vi "Trial v6.vi"(2 "error in (no error)":errorcluster, 3 "queue in":refnum<queue>, 4 "DDA":bool=TRUE) -> (0 "error out":errorcluster, 1 "queue out":refnum<queue>)   [LabVIEW 2017]
uses:
  <vilib>/Analysis/_algsub.llb/Real Vector Norm.vi
  <vilib>/Analysis/baseanly.llb/Real A x B.vi
  <vilib>/Analysis/baseanly.llb/Real Dot Product.vi
  <vilib>/Analysis/baseanly.llb/Outer Product.vi
  <vilib>/Analysis/baseanly.llb/Real Outer Product.vi
  <vilib>/robotics/Kinematics/Create Lie Group Matrix.vi
  SubVI/Global.vi
  <vilib>/Analysis/7linalg.llb/Create Special Matrix.vi
  <vilib>/Analysis/7linalg.llb/Create Special Real Matrix.vi
  <vilib>/Analysis/Matrix/Numeric/Multiply/Multiply.vi
  <vilib>/Analysis/Matrix/Numeric/Multiply/Multiply - RM,R.vi
  <vilib>/Analysis/Matrix/Numeric/Multiply/Multiply - R,RM.vi
  <vilib>/Analysis/Matrix/Numeric/Add/Add.vi
  <vilib>/Analysis/Matrix/Numeric/Add/Add - RM,RM.vi
  Control/Damping.ctl
  <vilib>/robotics/Kinematics/NI_Kinematics.lvlib
  <vilib>/Analysis/NI_AALBase.lvlib
  <vilib>/Analysis/NI_AALPro.lvlib
panel:
  in  "ACTION":dbl[](array[numeric])=[1.0, 0.5, -0.5, -1.0]
  in  "DELTAx":dbl=0.01
  in  "Algorithm Parameter":T1={"alpha Rbar"=0.1, "lambda w"=0.99, "lambda theta"=0.99, "alpha w"=0.1, "alpha theta"=0.1} {"alpha theta" scale=0.0..1.0; "alpha w" scale=0.0..1.0; "lambda theta" scale=0.0..1.0; "lambda w" scale=0.0..1.0; "alpha Rbar" scale=0.0..1.0}
  in  "Basis":enum16{"Polynomial", "Fourier"}(ring)
  in  "n":i32=2
  out "Guide":bool
  in  "DDA Wait (ms)":u32=1000
  in  "epsilon (deg)":dbl=5.0
  in  "Omega (deg/s)":dbl=10.0
  in  "Trial Wait (ms)":u32=10
  in  "RoM (deg)":dbl=75.0 format="%#_13g"
  out "Variable":T2={"state"=[1.0, 0.029510106398225495, 0.7899999999999947], "state'"=[1.0, 0.029510106398225495, 0.7899999999999947], "w"=[-0.776760178088027, 0.02290847510201797, -0.776760178088027, 0.0039017617832994905, -0.032305900148233264, 0.0039017617832994905, -0.008811939810442246, 0.006128296774504617, -0.008811939810442246, 0.08141039795404857, 0.024694708282895942, 0.08141039795404857, 0.000818616387278701, 0.013811079508305709, 0.000818616387278701, 0.007297971648903151, 0.00012749513787888267, 0.007297971648903151, 0.04749276911722675, 0.0020428849734649714, 0.04749276911722675, -0.0005749430419034135, 0.009106369563891898, -0.0005749430419034135, 0.004440396759161163, -0.00026837014810894707, 0.004440396759161163], "zw"=[46.90944570448865, 0.19066468600195396, 46.90944570448865, -0.7931005098682211, 5.860142075356345, -0.7931005098682211, 2.7017068020466164, -0.27486059004893465, 2.7017068020466164, 16.93934246409302, -0.551912667218565, 16.93934246409302, -0.5655566099588606, 2.5899820994142524, -0.5655566099588606, 1.2460084406100564, -0.1713251360039408, 1.2460084406100564, 9.289011953386677, -0.47204075792696587, 9.289011953386677, -0.4122416203188374, 1.437667453855831, -0.4122416203188374, 0.7051975708183595, -0.13015957998160824, 0.7051975708183595], "theta"=[1.4914571304587486e-15, 7.444904250698107e-17, 1.4914571304587486e-15, -4.739219774861162e-16, 6.634247906152909e-16, -4.739219774861162e-16, 7.576246728345865e-17, -1.7431691862520748e-17, 7.576246728345865e-17, 6.558028522386373e-17, 5.693079546893576e-16, 6.558028522386373e-17, 3.990875526750827e-17, -3.9273504773765236e-17, 3.990875526750827e-17, 2.459332078486038e-18, 1.1844914586165022e-17, 2.459332078486038e-18, 1.6785560810690787e-17, 4.0992884372049907e-17, 1.6785560810690787e-17, 1.547195777204608e-17, -1.8245201415855317e-17, 1.547195777204608e-17, 2.728657325438036e-18, -1.5522560327373708e-18, 2.728657325438036e-18, 25.646102280776066, 16.99493096232432, 25.646102280776066, 3.4822002128803744, 1.8527275230967626, 3.4822002128803744, 0.47573357341205397, 0.21371320352095907, 0.47573357341205397, -0.5264282474235465, -0.5422694989375832, -0.5264282474235465, -0.06394125843286388, -0.06344726999994278, -0.06394125843286388, -0.007905815409065703, -0.008246766308638343, -0.007905815409065703, 0.016635359284166797, 0.01856234594691108, 0.016635359284166797, 0.0019481630383850373, 0.0019346346383257145, 0.0019481630383850373, 0.00022262613770425934, 0.0002462738805832368, 0.00022262613770425934, -15.883327960756356, -27.94126620796533, -15.883327960756356, -1.4668314615111306, -3.9624707541982542, -1.4668314615111306, -0.1616174346023939, -0.5356497273885115, -0.1616174346023939, 0.5812202773533058, 0.5336991802087973, 0.5812202773533058, 0.06450129455154789, 0.06598340428988386, 0.06450129455154789, 0.008688278747498104, 0.007665438304981554, 0.008688278747498104, -0.021645624159105748, -0.015864851158712733, -0.021645624159105748, -0.0019966454372759715, -0.002037241101393498, -0.0019966454372759715, -0.0002749105366125961, -0.00020396807290514954, -0.0002749105366125961], "ztheta"=[7.054061451920969e-17, -3.9587003301846824e-16, 7.054061451920969e-17, 6.735802826201208e-18, -4.6286977384745565e-17, 6.735802826201208e-18, 1.393348122000214e-17, -2.2778836767459474e-17, 1.393348122000214e-17, -1.320687697955934e-16, 4.010916693070787e-17, -1.320687697955934e-16, -3.0638380335155074e-17, 3.0483525341288226e-17, -3.0638380335155074e-17, 1.0341705245027453e-17, -1.2480413093924516e-17, 1.0341705245027453e-17, 2.89630956686208e-17, -3.801392344852731e-17, 2.89630956686208e-17, 2.423591043688077e-17, -2.3809460948435052e-17, 2.423591043688077e-17, 4.616160753220477e-18, -4.795459759566049e-18, 4.616160753220477e-18, -2.910976576435246, -1.923969710656085, -2.910976576435246, -0.3974772560222368, -0.2077962325162933, -0.3974772560222368, -0.054121648119702236, -0.024130482735325663, -0.054121648119702236, 0.059512355276425906, 0.06158016230321163, 0.059512355276425906, 0.007261479780099875, 0.007188638739252933, 0.007261479780099875, 0.0008936446993227526, 0.0009399166521141767, 0.0008936446993227526, -0.0018547408233615288, -0.0021286028828297597, -0.0018547408233615288, -0.00022180803768472273, -0.0002182870264243828, -0.00022180803768472273, -2.4785505426840216e-05, -2.841860420413458e-05, -2.4785505426840216e-05, 1.8080184700730275, 3.160240158328639, 1.8080184700730275, 0.16194822643111972, 0.45396056921070077, 0.16194822643111972, 0.01843165528111534, 0.06070135065256019, 0.01843165528111534, -0.0662462980572756, -0.06004323366484613, -0.0662462980572756, -0.007289851049687639, -0.007508393437731105, -0.007289851049687639, -0.000997466379730686, -0.0008586521896839331, -0.000997466379730686, 0.0025324316646370623, 0.0017108705851870154, 0.0025324316646370623, 0.0002232616330359063, 0.00023382606595410158, 0.0002232616330359063, 3.261164823906294e-05, 2.1712455435348493e-05, 3.261164823906294e-05], "R"=0.34176612385999994, "Rbar"=-0.5362314277071021, "eligibility vector"=[0.0, 0.0, 0.0, 0.0, 0.0, 0.0, 0.0, 0.0, 0.0, 0.0, 0.0, 0.0, 0.0, 0.0, 0.0, 0.0, 0.0, 0.0, 0.0, 0.0, 0.0, 0.0, 0.0, 0.0, 0.0, 0.0, 0.0, 0.0, 0.0, 0.0, 0.0, 0.0, 0.0, 0.0, 0.0, 0.0, 0.0, 0.0, 0.0, 0.0, 0.0, 0.0, 0.0, 0.0, 0.0, 0.0, 0.0, 0.0, 0.0, 0.0, 0.0, 0.0, 0.0, 0.0, 0.0, 0.0, 0.0, 0.0, 0.0, 0.0, 0.0, 0.0, 0.0, 0.0, 0.0, 0.0, 0.0, 0.0, 0.0, 0.0, 0.0, 0.0, 0.0, 0.0, 0.0, 0.0, 0.0, 0.0, 0.0, 0.0, 0.0]} {"eligibility vector" format="%#_6f"; "ztheta" format="%#_6f"; "zw" format="%#_6f"; "Rbar" format="%#_6f"; "R" format="%#_6f"; "theta" format="%#_6f"; "w" format="%#_6f"}
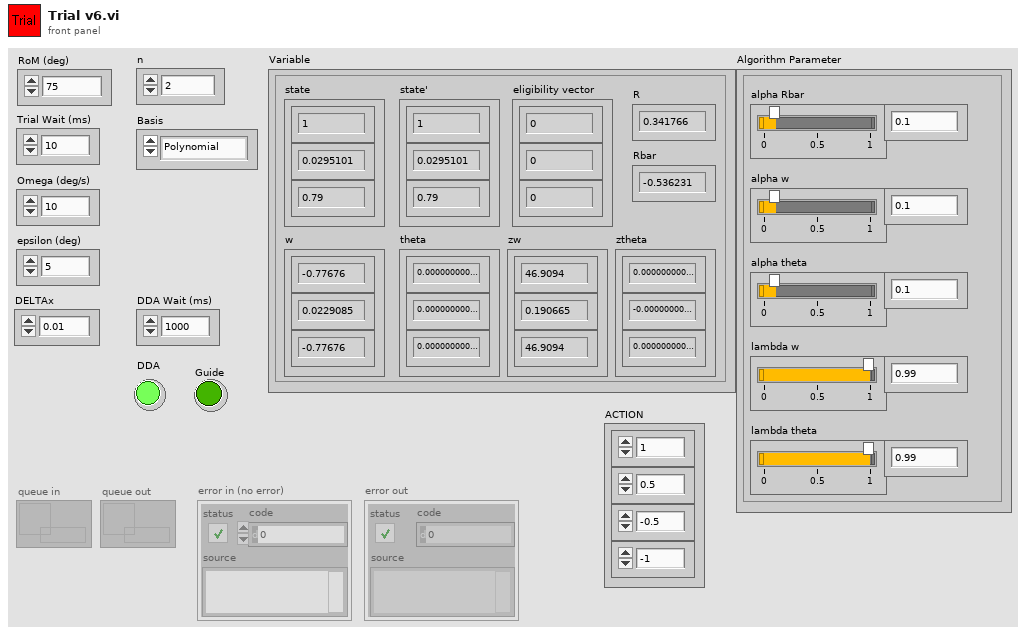
[diagram p1: front panel]
types:
  T1 = cluster{"alpha Rbar":dbl, "lambda w":dbl, "lambda theta":dbl, "alpha w":dbl, "alpha theta":dbl}
  T2 = cluster{"state":dbl[], "state'":dbl[], "w":dbl[], "zw":dbl[], "theta":dbl[], "ztheta":dbl[], "R":dbl, "Rbar":dbl, "eligibility vector":dbl[]}
  T3 = typedef "NI_Matrix.lvlib/RealMatrix.ctl" = dbl[][]
  T4 = typedef "Damping.ctl" = cluster{"Cx":dbl, "Cy":dbl, "Cz":dbl}
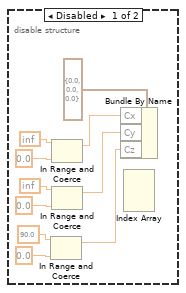
[diagram p2: hidden frame]
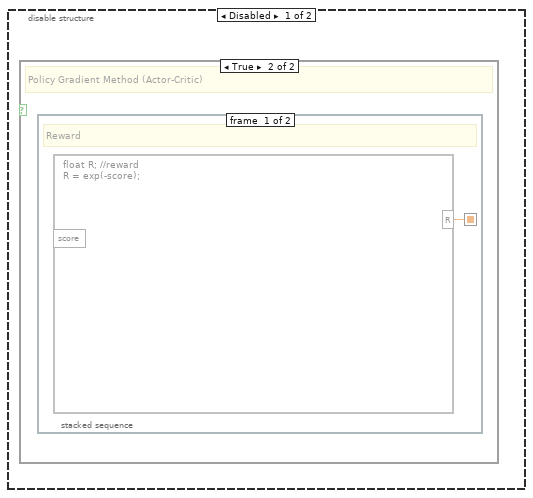
[diagram p3: hidden frame]
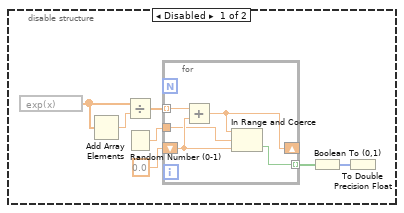
[diagram p6: hidden frame]
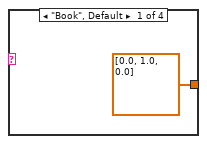
[diagram p9: hidden frame]
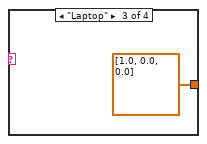
[diagram p10: hidden frame]
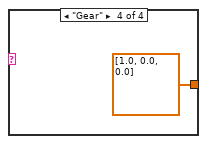
[diagram p11: hidden frame]
diagram:
  n1 = flat-sequence {
    tunnel: "DDA" -> [w11]
    tunnel: "queue in" -> [w10]
    tunnel: "error in (no error)" -> [w9]
    tunnel: [w8] -> w2
    tunnel: [w7] -> w1
    frame #0 {
      n2 = global read "Global.vi" "ADL"() -> (w14:string)
      n3 = case shown="True" w11 {
        tunnel: w10 -> [w16 w32]
        tunnel: w9 -> [w15 w31]
        tunnel: [w15 w29] -> w8
        tunnel: [w16 w30] -> w7
        frame False {
        }
        frame True {
          n4 = call "State.vi"() -> ("state"=w18:dbl[])  [unwired: 11 in]
          n5 = Build Array (concatenate)(w18, 0.0 ("element")) -> (w27:dbl[])
          n6 = call "Feature Vector.vi"("Basis"="Basis", "n"="n", "input"=w18) -> ("feature vector"=w36:dbl[])  [unwired: 8 in]
          n7 = call "Feature Vector.vi"("Basis"="Basis", "n"="n", "input"=w27) -> ("feature vector"=w24:dbl[])  [unwired: 8 in]
          n8 = Array Size(array=w36) -> (size(s)=w35:i32)
          n9 = Array Size(array=w24) -> (size(s)=w23:i32)
          n10 = Initialize Array(0.0 ("element"), w35) -> (w26:dbl[])
          n11 = Initialize Array(0.0 ("element"), w23) -> (w22:dbl[])
          n12 = Bundle By Name(cluster=T2 {"state"=[0.0, 0.0, 0.0], "state'"=[0.0, 0.0, 0.0], "w"=[0.0], "zw"=[0.0], "theta"=[0.0], "ztheta"=[0.0], "R"=0.0, "Rbar"=0.0, "eligibility vector"=[0.0]} ("Variable"), "state"=w18, "w"=w26, "zw"=w26, "theta"=w22, "ztheta"=w22, "Rbar"=0.0) -> (w19:T2)
          n13 = while {
            shift-right: [w38] -> _
            shift-left: w19 -> [w37]
            shift-right: [w42] -> w30
            shift-left: w32 -> [w44]
            shift-right: [w41] -> w29
            shift-left: w31 -> [w43]
            tunnel: "n" -> [w40]
            tunnel: "Basis" -> [w39]
            stop <- w46 stop-if-true
            n14 = local read "Guide"() -> (w45:bool)
            n15 = case shown="True" w45 {
              tunnel: w37 -> [w47 w60]
              tunnel: w44 -> [w49 w67]
              tunnel: w43 -> [w48 w66]
              tunnel: [w49 w65] -> w42
              tunnel: [w48 w64] -> w41
              tunnel: w40 -> [_ w62]
              tunnel: w39 -> [_ w61]
              tunnel: [w47 w56] -> w38
              frame False {
              }
              frame True {
                n16 = flat-sequence {
                  tunnel: w62 -> [w69]
                  tunnel: w61 -> [w68]
                  tunnel: w60 -> [w83]
                  tunnel: [w71] -> w59
                  tunnel: [w69] -> w53
                  tunnel: [w68] -> w50
                  tunnel: w59 -> [w113]
                  tunnel: [w113] -> w58
                  tunnel: [w112] -> w54
                  tunnel: w53 -> [w112]
                  tunnel: [w111] -> w51
                  tunnel: w50 -> [w111]
                  tunnel: w58 -> [w120]
                  tunnel: [w119] -> w57
                  tunnel: [w118] -> w55
                  tunnel: w54 -> [w118]
                  tunnel: [w117] -> w52
                  tunnel: w51 -> [w117]
                  tunnel: w57 -> [w124]
                  tunnel: [w123] -> w56
                  tunnel: w55 -> [w122]
                  tunnel: w52 -> [w121]
                  frame #0 {
                    # "Take Action"
                    n17 = Unbundle By Name(w83) -> ("state"=w70:dbl[], "theta"=w91:dbl[])
                    n18 = for {
                      tunnel: "ACTION" -> [w109] mode=indexing
                      tunnel: w70 -> [w110]
                      tunnel: w91 -> [w107]
                      tunnel: w69 -> [w106]
                      tunnel: w68 -> [w105]
                      tunnel: [w104] -> w90 mode=indexing
                      tunnel: [w103] -> w72 mode=indexing
                      n19 = Build Array (concatenate)(w110, w109) -> (w108:dbl[])
                      n20 = call "Feature Vector.vi"("Basis"=w105, "n"=w106, "input"=w108) -> ("feature vector"=w103:dbl[])  [unwired: 8 in]
                      n21 = call-poly <vilib>:"Dot Product.vi"("Y Vector"=w103, "X Vector"=w107) -> ("X * Y"=w104:dbl)  [unwired: 1 out]
                    }
                    n22 = Exponential(1:w90) -> (0:w88:dbl[])
                    n23 = Add Array Elements(numeric array=w88) -> (sum=w89:dbl)
                    n24 = Divide(x=w88, y=w89) -> (x/y=w79:dbl[])
                    n25 = Random Number (0-1)() -> (number: 0 to 1=w86:dbl)
                    n26 = for {
                      tunnel: w79 -> [w102] mode=indexing
                      shift-right: [w98] -> _
                      shift-left: 0.0 -> [w101]
                      tunnel: w86 -> [w100]
                      tunnel: [w97] -> w85
                      i -> [w97]
                      stop <- w99 stop-if-true
                      n27 = Add(x=w102, y=w101) -> (x+y=w98:dbl)
                      n28 = In Range and Coerce(upper limit=w98, x=w100, lower limit=w101) -> (In Range?=w99:bool)  [unwired: 1 out]
                    }
                    n29 = Index Array(array="ACTION", index=w85) -> (element=w82:dbl)
                    n30 = Build Array (concatenate)(w70, w82) -> (w81:dbl[])
                    n31 = call "Action.vi"("DELTAx"="DELTAx", "action"=w82) -> ()  [unwired: 10 in]
                    n32 = call "Feature Vector.vi"("Basis"=w68, "n"=w69, "input"=w81) -> ("feature vector"=w78:dbl[])  [unwired: 8 in]
                    n33 = Array Size(array=w78) -> (size(s)=w77:i32)
                    n34 = Initialize Array(0.0 ("element"), w77) -> (w75:dbl[])
                    n35 = for {
                      tunnel: w79 -> [w96] mode=indexing
                      shift-right: [w93] -> w74
                      shift-left: w75 -> [w95]
                      tunnel: w72 -> [w92] mode=indexing
                      n36 = Multiply(x=w96, y=w92) -> (x*y=w94:dbl[])
                      n37 = Add(x=w95, y=w94) -> (x+y=w93:dbl[])
                    }
                    n38 = Subtract(x=w78, y=w74) -> (x-y=w73:dbl[])
                    n39 = Bundle By Name(cluster=w83, "eligibility vector"=w73) -> (w71:T2)
                  }
                  frame #1 {
                    # "Wait"
                    n40 = Wait (ms)(milliseconds to wait="DDA Wait (ms)") -> ()  [unwired: 1 out]
                  }
                  frame #2 {
                    # "Observe"
                    n41 = call "State.vi"() -> ("state"=w116:dbl[])  [unwired: 11 in]
                    n42 = call "Reward.vi"() -> ("reward"=w115:dbl)  [unwired: 11 in]
                    n43 = Bundle By Name(cluster=w120, "state'"=w116, "R"=w115) -> (w119:T2)
                  }
                  frame #3 {
                    # "Algorithm"
                    n44 = call "Algorithm.vi"("Algorithm Parameter"="Algorithm Parameter", "Basis"=w121, "n"=w122, "Variable"=w124) -> ("Variable"=w123:T2)  [unwired: 7 in]
                  }
                }
                n45 = Enqueue Element(queue=w67, element="", error in (no error)=w66) -> (queue out=w65:refnum<queue>, error out=w64:errorcluster)  [unwired: 1 in, 1 out]
              }
            }
            n46 = global read "Global.vi" "Stop"() -> (w46:bool)
            "Variable" <- w37
          }
        }
      }
      n47 = case shown="\"Pitcher\"" w14 {
        tunnel: [dbl[] [0.0, 1.0, 0.0] dbl[] [0.0, -1.0, 0.0] dbl[] [1.0, 0.0, 0.0] dbl[] [1.0, 0.0, 0.0]] -> w12
        frame "Book", Default {
        }
        frame "Pitcher" {
        }
        frame "Laptop" {
        }
        frame "Gear" {
        }
      }
      n48 = expression code="(x/180.0)*pi" "degrees to radians"("RoM (deg)") -> (w6:dbl)
      n49 = while {
        tunnel: w6 -> [w134]
        tunnel: w12 -> [w132]
        i -> [w136]
        stop <- w135 stop-if-true
        # "1 Trial"
        n50 = flat-sequence {
          tunnel: w136 -> [w150]
          tunnel: w134 -> [w144]
          tunnel: [w142] -> w133
          tunnel: w132 -> [w140]
          tunnel: [w138] -> w131
          tunnel: [w137] -> w130
          frame #0 {
            w145 = 0.0 ("f")
            n51 = Negate(x=w140) -> (-x=w139:dbl[])
            n52 = Quotient & Remainder(x=w150, y=2) -> (x-y*floor(x/y)=w148:i32)  [unwired: 1 out]
            n53 = Equal To 0?(x=w148) -> (x = 0?=w141:bool)
            n54 = Select(t=w145, s=w141, f=w144) -> (s? t:f=w143:dbl)
            n55 = Select(t=w144, s=w141, f=w145) -> (s? t:f=w146:dbl)
            n56 = Select(t=w140, s=w141, f=w139) -> (s? t:f=w138:dbl[])
            n57 = call <vilib>:"Angle Vector to Rotation Matrix.vi"("vector"=w140, "angle"=w143) -> ("rotation matrix"=w142:T3)
            n58 = call <vilib>:"Angle Vector to Rotation Matrix.vi"("vector"=w140, "angle"=w146) -> ("rotation matrix"=w147:T3)
            n59 = call <vilib>:"Rotation Matrix to Roll Pitch Yaw.vi"("rotation matrix"=w147) -> ("angles"=w137:cluster{"roll":dbl, "pitch":dbl, "yaw":dbl})
          }
        }
        n60 = while {
          shift-right: [w154] -> _
          shift-left: w133 -> [w155]
          tunnel: w131 -> [w156]
          tunnel: w130 -> [w151]
          stop <- w152 stop-if-true
          # "1/2 Trial"
          n61 = Wait (ms)(milliseconds to wait="Trial Wait (ms)") -> ()  [unwired: 1 out]
          n62 = flat-sequence {
            tunnel: w156 -> [w183]
            tunnel: w155 -> [w182]
            tunnel: [w180] -> w154
            tunnel: "Trial Wait (ms)" -> [w179]
            tunnel: w151 -> [w167]
            tunnel: [w161] -> w152
            frame #0 {
              n63 = To Double Precision Float(number=w179) -> (double precision float=w178:dbl)
              n64 = call <vilib>:"Rotation Matrix to Roll Pitch Yaw.vi"("rotation matrix"=w182) -> ("angles"=w166:cluster{"roll":dbl, "pitch":dbl, "yaw":dbl})
              n65 = global read "Global.vi" "Object"() -> (w173:cluster{"roll":dbl, "pitch":dbl, "yaw":dbl})
              n66 = global write "Global.vi" "Guide"(w166) -> ()
              n67 = Subtract(x=w167, y=w166) -> (x-y=w168:cluster{"roll":dbl, "pitch":dbl, "yaw":dbl})
              n68 = expression code="(x/180.0)*pi" "degrees to radians"("Omega (deg/s)") -> (w175:dbl)
              n69 = expression code="x/1000"(w178) -> (w177:dbl)
              n70 = Subtract(x=w167, y=w173) -> (x-y=w172:cluster{"roll":dbl, "pitch":dbl, "yaw":dbl})
              n71 = Cluster To Array(cluster=w168) -> (array=w169:dbl[])
              n72 = expression code="(x/180.0)*pi" "degrees to radians"("epsilon (deg)") -> (w158:dbl)
              n73 = Multiply(x=w177, y=w175) -> (x*y=w174:dbl)
              n74 = call-poly <vilib>:"Vector Norm.vi"("Input Vector"=w169) -> ("norm"=w159:dbl)  [unwired: 9 in, 1 out]
              n75 = Cluster To Array(cluster=w172) -> (array=w171:dbl[])
              n76 = global read "Global.vi" "Playback"() -> (w165:bool)
              n77 = Greater Or Equal?(x=w159, y=w158) -> (x >= y?=w157:bool)
              n78 = call-poly <vilib>:"Vector Norm.vi"("Input Vector"=w171) -> ("norm"=w170:dbl)  [unwired: 9 in, 1 out]
              n79 = global read "Global.vi" "Stop"() -> (w163:bool)
              n80 = Less?(x=w170, y=w158) -> (x < y?=w162:bool)
              n81 = call <vilib>:"Angle Vector to Rotation Matrix.vi"("vector"=w183, "angle"=w174) -> ("rotation matrix"=w181:T3)
              n82 = And(x=w157, y=w165) -> (x .and. y?=w164:bool)
              "Guide" <- w164
              n83 = Or(x=w163, y=w162) -> (x .or. y?=w161:bool)
              n84 = case shown="True" w164 {
                tunnel: w182 -> [w184 w187]
                tunnel: w181 -> [_ w186]
                tunnel: [w184 w185] -> w180
                frame False {
                }
                frame True {
                  n85 = call-poly <vilib>:"A x B.vi"("B"=w186, "A"=w187) -> ("A x B"=w185:T3)  [unwired: 1 out]
                }
              }
            }
          }
        }
        n86 = global read "Global.vi" "Stop"() -> (w135:bool)
      }
    }
  }
  n87 = disable-structure shown="Enabled" {
    frame Disabled {
      n88 = In Range and Coerce(upper limit=90.0, lower limit=0.0) -> (coerced(x)=w197:dbl)  [unwired: 1 in, 1 out]
      n89 = In Range and Coerce(upper limit=inf, lower limit=0.0) -> (coerced(x)=w195:dbl)  [unwired: 1 in, 1 out]
      n90 = In Range and Coerce(upper limit=inf, lower limit=0.0) -> (coerced(x)=w196:dbl)  [unwired: 1 in, 1 out]
      n91 = Bundle By Name(cluster=T4 {"Cx"=0.0, "Cy"=0.0, "Cz"=0.0} ("State"), "Cx"=w195, "Cy"=w196, "Cz"=w197) -> ()  [unwired: 1 out]
      n92 = Index Array() -> ()  [unwired: 4 in, 3 out]
    }
    frame Enabled {
    }
  }
  n93 = disable-structure shown="Enabled" {
    frame Disabled {
      n94 = expression code="exp(x)"() -> (w200:dbl[])  [unwired: 1 in]
      n95 = Add Array Elements(numeric array=w200) -> (sum=w201:dbl)
      n96 = Divide(x=w200, y=w201) -> (x/y=w198:dbl[])
      n97 = Random Number (0-1)() -> (number: 0 to 1=w202:dbl)
      n98 = for {
        shift-right: [w208] -> _
        shift-left: 0.0 -> [w209]
        tunnel: w202 -> [w207]
        tunnel: [w206] -> w203 mode=indexing
        tunnel: w198 -> [w205] mode=indexing
        n99 = Add(x=w205, y=w209) -> (x+y=w208:dbl)
        n100 = In Range and Coerce(upper limit=w208, x=w207, lower limit=w209) -> (In Range?=w206:bool)  [unwired: 1 out]
      }
      n101 = Boolean To (0,1)(Boolean=w203) -> (0, 1=w204:i16[])
      n102 = To Double Precision Float(number=w204) -> ()  [unwired: 1 out]
    }
    frame Enabled {
    }
  }
  n103 = disable-structure shown="Enabled" {
    frame Disabled {
      n104 = case shown="True" {
        selector: _ -> [_ _]
        frame False {
        }
        frame True {
          # "Policy Gradient Method (Actor-Critic)"
          n105 = stacked-sequence {
            seq-local: [w210 _] -> [_ _]
            frame #0 {
              # "Reward"
              n106 = formula code="float R; //reward\nR = exp(-score);"() -> ("R"=w210:dbl)  [unwired: 1 in]
            }
            frame #1 {
            }
          }
        }
      }
    }
    frame Enabled {
    }
  }
  "error out" <- w2
  "queue out" <- w1
